vi "PH_GUI.set U32 GUI object.vi"(0 "Caption [Empty]":string, 1 "Visible (True)":bool=TRUE, 2 "U32 Ref":refnum<vi>, 3 "Value":u32, 4 "Blinking (false)":bool, 5 "error in (no error)":errorcluster, 7 "Tip Strip [Empty]":string, 9 "Disabled (Enabled)":T1(ring)) -> (19 "error out":errorcluster)   [LabVIEW 2014, in "PH_Common.lvlib"]
doc: "Sets value and more for the referenced GUI object."
uses:
  PH_Common.lvlib
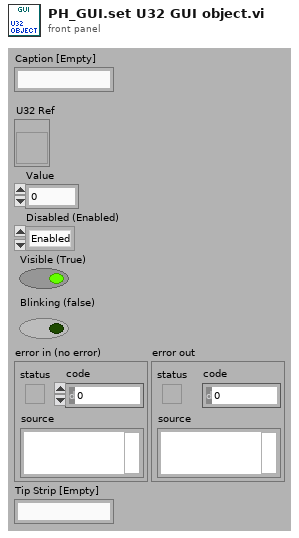
[diagram p1: front panel]
types:
  T1 = enum8{"Enabled", "Disabled", "Disabled and Grayed Out"}
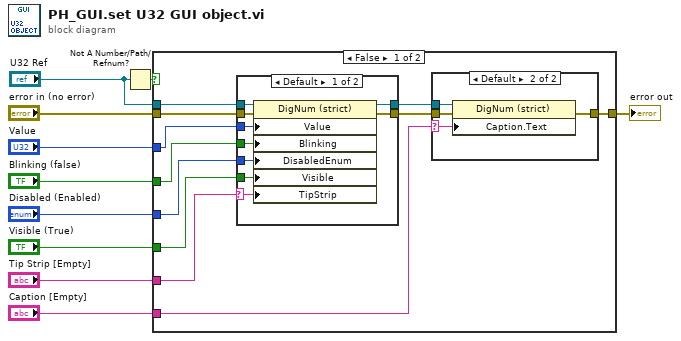
[diagram p0: block diagram]
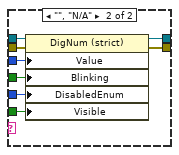
[diagram p3: hidden frame]
diagram:
  n1 = Not A Number/Path/Refnum?(number/path/refnum="U32 Ref") -> (NaN/Path/Refnum?=w9:bool)
  n2 = case shown="False" w9 {
    tunnel: "error in (no error)" -> [w17 w44]
    tunnel: "U32 Ref" -> [w18 _]
    tunnel: "Value" -> [w19 _]
    tunnel: "Blinking (false)" -> [w20 _]
    tunnel: [w13 w44] -> w6
    tunnel: "Tip Strip [Empty]" -> [w14 _]
    tunnel: "Disabled (Enabled)" -> [w16 _]
    tunnel: "Visible (True)" -> [w15 _]
    tunnel: "Caption [Empty]" -> [w11 _]
    frame False {
      n3 = case shown="Default" w14 {
        selector: w14 -> [w29 _]
        tunnel: [w28 w43] -> w21
        tunnel: w20 -> [w35 w42]
        tunnel: w19 -> [w34 w41]
        tunnel: w18 -> [w33 w40]
        tunnel: w17 -> [w32 w39]
        tunnel: w16 -> [w31 w38]
        tunnel: w15 -> [w30 w37]
        tunnel: [w27 w36] -> w12
        frame Default {
          n4 = property class="DigNum (strict)"(reference=w33, error in=w32, "Value"=w34, "Blinking"=w35, "DisabledEnum"=w31, "Visible"=w30, "TipStrip"=w29) -> (reference out=w27:refnum<vi>, error out=w28:errorcluster)
        }
        frame "", "N/A" {
          n5 = property class="DigNum (strict)"(reference=w40, error in=w39, "Value"=w41, "Blinking"=w42, "DisabledEnum"=w38, "Visible"=w37) -> (reference out=w36:refnum<vi>, error out=w43:errorcluster)
        }
      }
      n6 = case shown="Default" w11 {
        selector: w11 -> [_ w23]
        tunnel: w21 -> [w22 w26]
        tunnel: [w22 w25] -> w13
        tunnel: w12 -> [_ w24]
        frame "", "N/A" {
        }
        frame Default {
          n7 = property class="DigNum (strict)"(reference=w24, error in=w26, "Caption.Text"=w23) -> (error out=w25:errorcluster)  [unwired: 1 out]
        }
      }
    }
    frame True {
    }
  }
  "error out" <- w6
